vi "Get AO DMA Depth.vi"(8 "error in (no error)":errorcluster, 10 "DMA Depth In":u32[](array[numeric]), 11 "Action":enum16{"Get", "Set"}(ring)) -> (0 "error out":errorcluster, 3 "DMA Depth Out":u32[](array[numeric]))   [LabVIEW 2021]
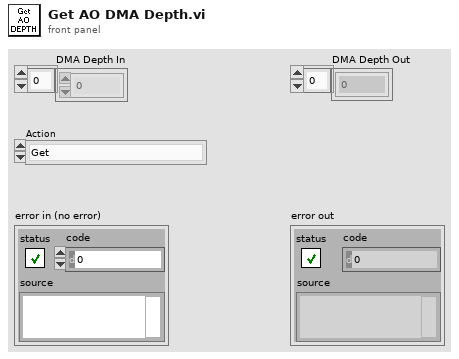
[diagram p1: front panel]
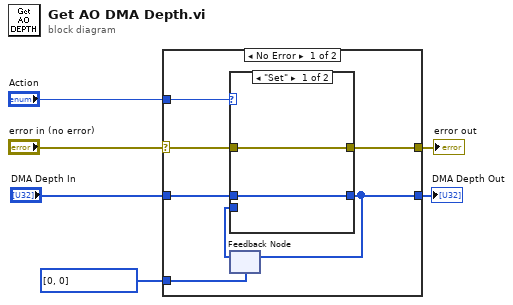
[diagram p0: block diagram]
diagram:
  n1 = case shown="No Error" "error in (no error)" {
    selector: "error in (no error)" -> [w8 w18]
    tunnel: "Action" -> [w12 _]
    tunnel: "DMA Depth In" -> [w11 _]
    tunnel: u32[] [0, 0] -> [w10 w19]
    tunnel: [w9 w18] -> w5
    tunnel: [w7 w19] -> w1
    frame No Error {
      n2 = feedback #1(w10) -> (w13:u32[])
      n3 = case shown="\"Set\"" w12 {
        tunnel: [w14 w16] -> w7
        tunnel: w13 -> [_ w16]
        tunnel: w11 -> [w14 _]
        tunnel: w8 -> [w15 w17]
        tunnel: [w15 w17] -> w9
        frame "Set" {
        }
        frame "Get" {
        }
      }
      n4 = feedback-in #1(w7) -> ()
    }
    frame Error {
    }
  }
  "error out" <- w5
  "DMA Depth Out" <- w1
